vi "modify tag.vi"(4 "original tag name":string, 5 "Number of Elements":u32=1, 6 "original network path":string, 7 "eip tag types":T1, 8 "error in":errorcluster, 9 "Tag Name":string, 10 "Network Path":string, 11 "EIP Tags configuration in":refnum<class "EIP Tags Configuration.lvclass">) -> (0 "error out":errorcluster, 2 "removed channels":refnum<class "EIP Tags Channel.lvclass">[](array[class]), 3 "EIP Tags configuration out":refnum<class "EIP Tags Configuration.lvclass">)   [LabVIEW 2013, in "EIP Tags Configuration.lvclass"]
uses:
  EIP Tags Configuration.lvclass
  eip tag types.ctl
  channel/EIP Tags Channel.lvclass
  EIP Tags Configuration.lvclass/EIP Tags Configuration.ctl
  channel/EIP Tags Channel.lvclass/EIP Tags Channel.ctl
  <vilib>/NI/Tag Bus/tag/tag descriptor.lvclass/tag descriptor.ctl
  channel/Write EIP Tag UUID.vi
  <vilib>/NI/Tag Bus/tag/write data type.vi
  channel/Read element.vi
  channel/Read EIP Tag UUID.vi
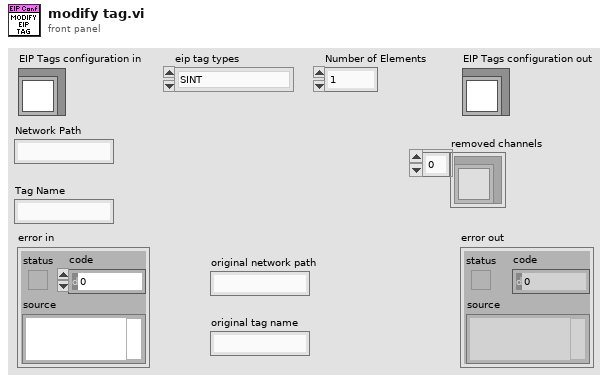
[diagram p1: front panel]
types:
  T1 = typedef "EIP Tags Configuration.lvclass/eip tag types.ctl" = enum16{"SINT", "INT", "DINT", "REAL", "BOOL", "STRING"}
  T2 = typedef "EIP Tags Configuration.lvclass/eip tag definition.ctl" = cluster{"eip tag types":T1, "unique tag name":string, "Number of Elements":u32}
  T3 = typedef "tag bus.lvlib/tag descriptor.lvclass/Data Type.ctl" = enum16{"Double", "Single", "I64", "I32", "I16", "I8", "U64", "U32", "U16", "U8", "Boolean", "String", "Array of Double", "Array of Single", "Array of I64", "Array of I32", "Array of I16", "Array of I8", "Array of U64", "Array of U32", "Array of U16", "Array of U8", "Array of Boolean", "Array of String"}
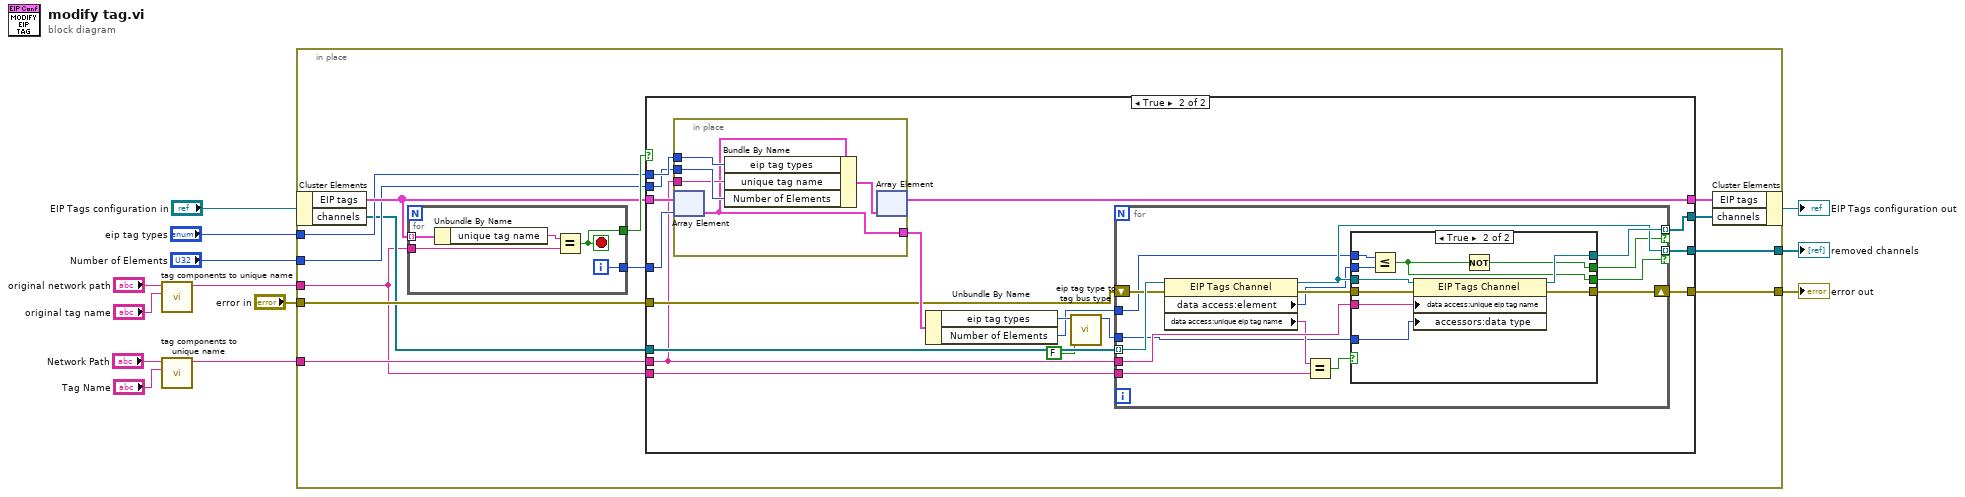
[diagram p0: block diagram]
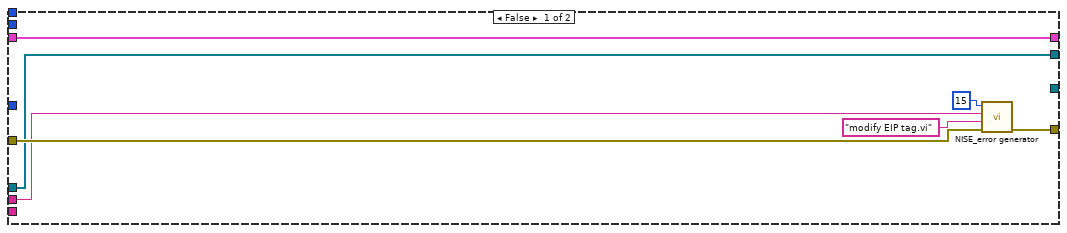
[diagram p2: hidden frame]
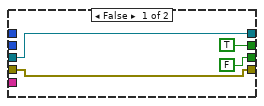
[diagram p3: hidden frame]
diagram:
  n1 = call "tag components to unique name.vi"("Tag Name"="original tag name", "Network Path"="original network path") -> ("unique name"=w2:string)  [unwired: 9 in]
  n2 = call "tag components to unique name.vi"("Tag Name"="Tag Name", "Network Path"="Network Path") -> ("unique name"=w8:string)  [unwired: 9 in]
  n3 = in-place {
    in-place-border: "error in" -> [w24]
    in-place-border: w8 -> [w21]
    in-place-border: [w25] -> w7
    in-place-border: "eip tag types" -> [w20]
    in-place-border: "Number of Elements" -> [w19]
    in-place-border: w2 -> [w15]
    in-place-border: [w14] -> w1
    n4 = in-place-cluster #1("EIP Tags configuration in") -> ("EIP tags"=w22:T2[], "channels"=w17:refnum<class "EIP Tags Channel.lvclass">[])
    n5 = for {
      tunnel: w22 -> [w89] mode=indexing
      tunnel: w15 -> [w87]
      tunnel: [w86] -> w26
      tunnel: [w85] -> w18
      i -> [w85]
      stop <- w86 stop-if-true
      n6 = Unbundle By Name(w89) -> ("unique tag name"=w88:string)
      n7 = Equal?(x=w88, y=w87) -> (x = y?=w86:bool)
    }
    n8 = case shown="True" w26 {
      tunnel: [w33 w40] -> w25
      tunnel: w24 -> [w32 w43]
      tunnel: [w30 w49] -> w23
      tunnel: w22 -> [w30 w50]
      tunnel: w21 -> [w29 w41]
      tunnel: w20 -> [_ w47]
      tunnel: w19 -> [_ w46]
      tunnel: w18 -> [_ w48]
      tunnel: w17 -> [w27 w44]
      tunnel: [w27 w39] -> w16
      tunnel: w15 -> [_ w42]
      tunnel: [_ w38] -> w14
      frame False {
        n9 = call <vilib>:"NISE_error generator.vi"("error in"=w32, "source"="modify EIP tag.vi", "append error message"=w29, "error code (0)"=15) -> ("error out"=w33:errorcluster)  [unwired: 5 in]
      }
      frame True {
        n10 = in-place {
          in-place-border: w47 -> [w83]
          in-place-border: w46 -> [w82]
          in-place-border: w41 -> [w81]
          in-place-border: [w80] -> w45
          n11 = in-place-array #2(w50, w48) -> (w80:T2)
          n12 = Bundle By Name(cluster=w80, "eip tag types"=w83, "unique tag name"=w81, "Number of Elements"=w82) -> (w84:T2)
          n13 = in-place-array #2(w84) -> (w49:T2[])  [unwired: 1 out]
        }
        n14 = Unbundle By Name(w45) -> ("eip tag types"=w37:T1, "Number of Elements"=w35:u32)
        n15 = call "eip tag type to tag bus type.vi"("array?"=FALSE, "eip tag types"=w37) -> ("data type"=w36:T3)  [unwired: 9 in]
        n16 = for {
          tunnel: w44 -> [w65] mode=indexing
          shift-right: [w62] -> w40
          shift-left: w43 -> [w64]
          tunnel: w42 -> [w61]
          tunnel: w41 -> [w59]
          tunnel: [w57] -> w39 mode=indexing if=w54
          tunnel: [w56] -> w38 mode=indexing if=w55
          tunnel: w36 -> [w52]
          tunnel: w35 -> [w51]
          n17 = property class="EIP Tags Channel"(reference=w65, error in=w64) -> (reference out=w56:refnum<class "EIP Tags Channel.lvclass">, error out=w63:errorcluster, "data access:element"=w53:i32, "data access:unique eip tag name"=w58:string)
          n18 = Equal?(x=w58, y=w61) -> (x = y?=w60:bool)
          n19 = case shown="True" w60 {
            tunnel: w56 -> [w69 w79]
            tunnel: w63 -> [w68 w78]
            tunnel: [w68 w77] -> w62
            tunnel: w59 -> [_ w76]
            tunnel: [w69 w75] -> w57
            tunnel: [FALSE w71] -> w55
            tunnel: [TRUE w70] -> w54
            tunnel: w53 -> [_ w72]
            tunnel: w52 -> [_ w74]
            tunnel: w51 -> [_ w73]
            frame False {
            }
            frame True {
              n20 = Less Or Equal?(x=w73, y=w72) -> (x <= y?=w71:bool)
              n21 = property class="EIP Tags Channel"(reference=w79, error in=w78, "data access:unique eip tag name"=w76, "accessors:data type"=w74) -> (reference out=w75:refnum<class "EIP Tags Channel.lvclass">, error out=w77:errorcluster)
              n22 = Not(x=w71) -> (.not. x?=w70:bool)
            }
          }
        }
      }
    }
    n23 = in-place-cluster #1("EIP tags"=w23, "channels"=w16) -> (→"EIP Tags configuration out":refnum<class "EIP Tags Configuration.lvclass">)
  }
  "error out" <- w7
  "removed channels" <- w1
